vi "getWifiMode.vi"(8 "error":errorcluster, 11 "connection ID":refnum<k5>) -> (0 "error out":errorcluster, 2 "mode":i32, 3 "connection ID out":refnum<k5>)   [LabVIEW 2016, in "amc_api.lvlib"]
doc: "Gets the operation mode of the WiFi adapter."
uses:
  amc_api.lvlib
panel:
  out "jsonRespIn":string
  out "JSON-response":string="{\"jsonrpc\":\"2.0\",\"method\":\"\",\"params\":[5,1.245,true,\"name\"],\"id\":\"1\"}"
  out "JSON request":string
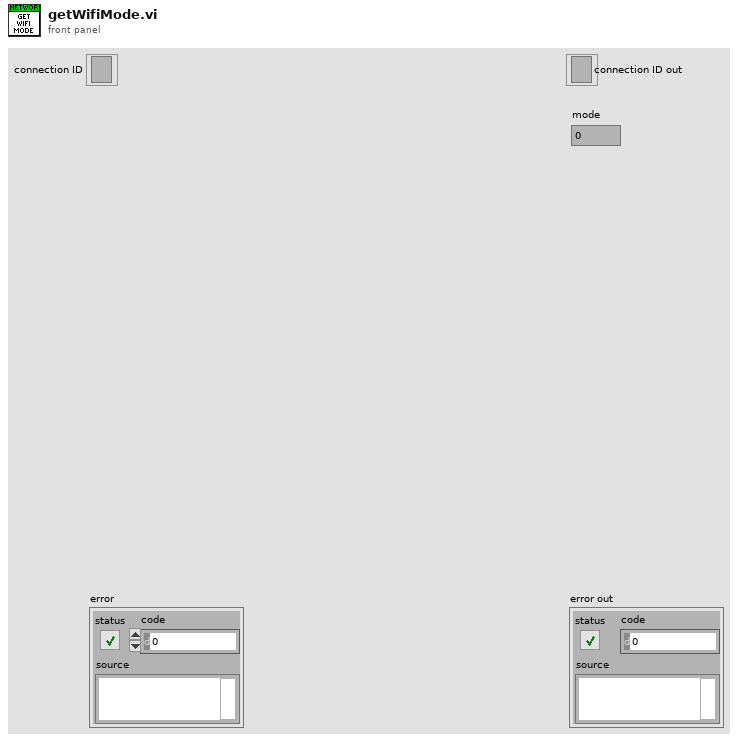
[diagram p1: front panel]
types:
  T1 = cluster{"jsonrpc":string, "method":string, "params":string[], "id":string, "api":i32, "pid":string}
  T2 = enum16{"Standard", "Buffered", "CRLF", "Immediate"}
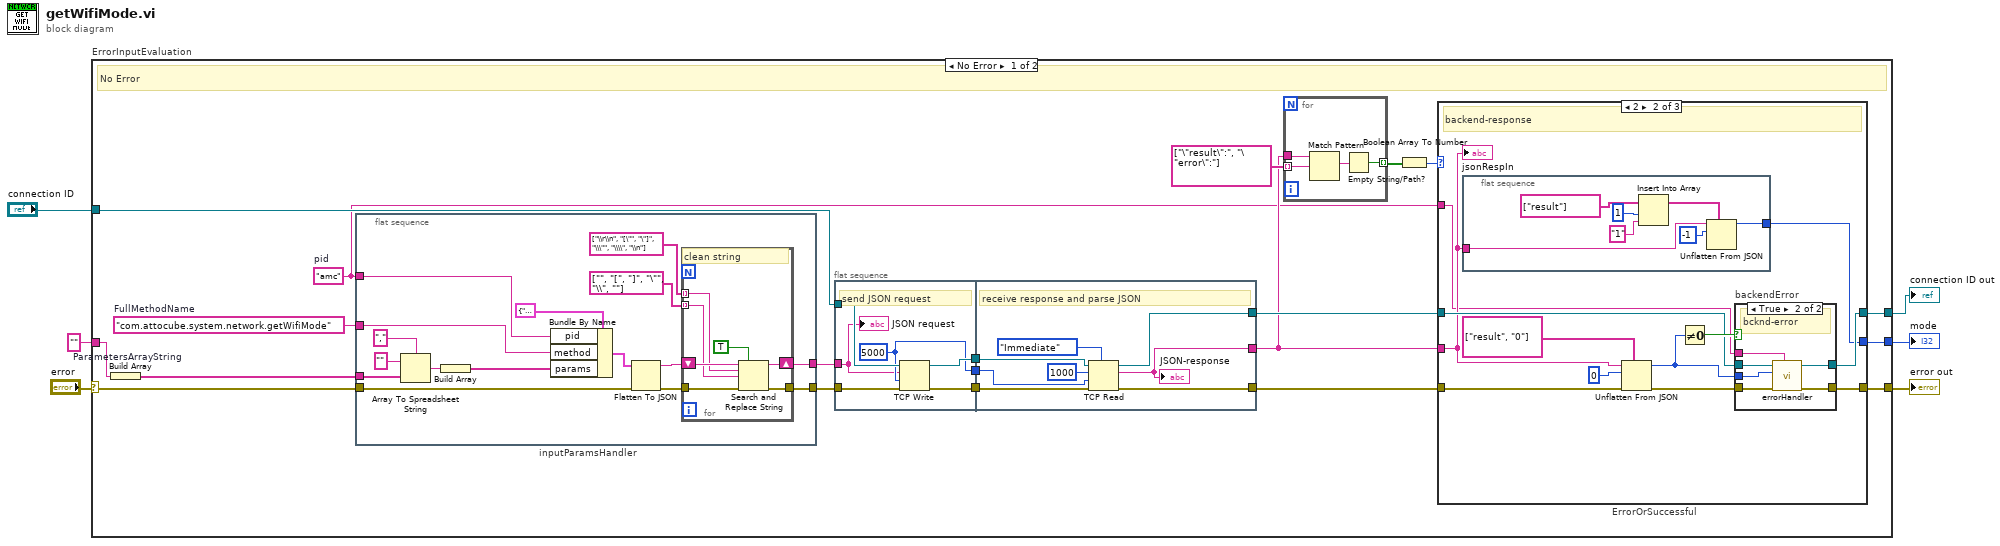
[diagram p0: block diagram]
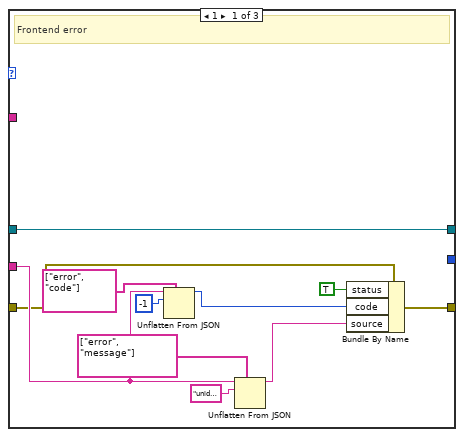
[diagram p2: hidden frame]
diagram:
  n1 = case "ErrorInputEvaluation" shown="No Error" "error" {
    selector: "error" -> [w13 w108]
    tunnel: "connection ID" -> [w23 w109]
    tunnel: [w15 w108] -> w5
    tunnel: [w16 w109] -> w4
    tunnel: "" -> [w8 _]
    tunnel: [w7 _] -> w1
    frame No Error {
      w9 = "amc"  # pid
      w14 = "com.attocube.system.network.getWifiMode"  # FullMethodName
      # "No Error"
      n2 = Build Array "ParametersArrayString"(w8) -> (w12:string[])
      n3 = flat-sequence "inputParamsHandler" {
        tunnel: [w32] -> w11
        tunnel: w12 -> [w38]
        tunnel: w13 -> [w37]
        tunnel: [w34] -> w10
        tunnel: w14 -> [w28]
        tunnel: w9 -> [w27]
        frame #0 {
          n4 = Array To Spreadsheet String(delimiter (Tab)=",", array=w38, 3:"" ("format string")) -> (spreadsheet string=w40:string)
          n5 = Build Array "Build Array"(w40) -> (w29:string[])
          n6 = Bundle By Name(cluster=T1 {"jsonrpc"="2.0", "method"="com.attocube.amc.res.setRESReadOutFreq", "params"=[], "id"="1", "api"=2, "pid"=""}, "pid"=w27, "method"=w28, "params"=w29) -> (w39:T1)
          n7 = Flatten To JSON(anything=w39, error in (no error)=w37) -> (JSON string=w33:string, 11:w35:errorcluster)  [unwired: 1 in]
          n8 = for {
            tunnel: string[] ["\\r\\n", "[\"", "\"]", "\\\"", "\\\\", "\\n"] ("search string") -> [w46] mode=indexing
            tunnel: string[] ["", "[", "]", "\"", "\\", ""] ("replace string (\"\")") -> [w45] mode=indexing
            shift-right: [w48] -> w32
            shift-left: w33 -> [w47]
            tunnel: w35 -> [w44]
            tunnel: [w43] -> w34
            # "clean string"
            n9 = Search and Replace String(replace all?=TRUE ("replace all? (F)"), input string=w47, search string=w46, replace string=w45, error in=w44) -> (result string=w48:string, error out=w43:errorcluster)  [unwired: 3 in, 2 out]
          }
        }
      }
      n10 = flat-sequence {
        tunnel: w23 -> [w99]
        tunnel: [w97] -> w26
        tunnel: [w98] -> w25
        tunnel: w10 -> [w94]
        tunnel: [w96] -> w24
        tunnel: w11 -> [w95]
        tunnel: [w103] -> w19
        tunnel: w26 -> [w105]
        tunnel: w25 -> [w104]
        tunnel: [w101] -> w18
        tunnel: w24 -> [w102]
        tunnel: [w100] -> w17
        frame #0 {
          w96 = 5000 ("timeout ms (25000)")
          # "send JSON request"
          n11 = TCP Write(connection ID=w99, data in=w95, error in (no error)=w94, 9:w96) -> (connection ID out=w97:refnum<k5>, error out=w98:errorcluster)  [unwired: 1 out]
          "JSON request" <- w95
        }
        frame #1 {
          # "receive response and parse JSON"
          n12 = TCP Read(connection ID=w105, bytes to read=1000, error in (no error)=w104, 7:T2."Immediate" ("mode (standard)"), 9:w102) -> (connection ID out=w103:refnum<k5>, data out=w100:string, error out=w101:errorcluster)
          "JSON-response" <- w100
        }
      }
      n13 = for {
        tunnel: string[] ["\"result\":", "\"error\":"] ("path") -> [w52] mode=indexing
        tunnel: [w50] -> w21 mode=indexing
        tunnel: w17 -> [w53]
        n14 = Match Pattern(string=w53, regular expression=w52) -> (match substring=w51:string)  [unwired: 1 in, 3 out]
        n15 = Empty String/Path?(string/path=w51) -> (empty?=w50:bool)
      }
      n16 = Boolean Array To Number(Boolean array=w21) -> (number=w20:u32)
      n17 = case "ErrorOrSuccessful" shown="2" w20 {
        tunnel: w17 -> [w56 w67 _]
        tunnel: w19 -> [w54 w70 w93]
        tunnel: [w54 w69 w93] -> w16
        tunnel: [w57 w68 w92] -> w15
        tunnel: w18 -> [w55 w71 w92]
        tunnel: w9 -> [_ w66 _]
        tunnel: [_ w65 _] -> w7
        frame 1 {
          # "Frontend error"
          n18 = Unflatten From JSON(path=string[] ["error", "code"], JSON string=w56, type and defaults=-1) -> (value=w63:i32)  [unwired: 4 in, 1 out]
          n19 = Unflatten From JSON(path=string[] ["error", "message"], JSON string=w56, type and defaults="unidentified error") -> (value=w64:string)  [unwired: 4 in, 1 out]
          n20 = Bundle By Name(cluster=w55, "status"=TRUE, "code"=w63, "source"=w64) -> (w57:errorcluster)
        }
        frame 2 {
          # "backend-response"
          n21 = flat-sequence "out_integer" {
            tunnel: w67 -> [w79]
            tunnel: [w77] -> w65
            frame #0 {
              n22 = Insert Into Array(array=string[] ["result"] ("path"), index=1, new element="1" ("idx")) -> (w81:string[])
              n23 = Unflatten From JSON(path=w81, JSON string=w79, type and defaults=-1 ("index")) -> (value=w77:i32)  [unwired: 4 in, 1 out]
            }
          }
          n24 = Unflatten From JSON(path=string[] ["result", "0"], JSON string=w67, type and defaults=0, error in (no error)=w71) -> (value=w76:i32, error out=w74:errorcluster)  [unwired: 3 in]
          n25 = Not Equal To 0?(x=w76) -> (x != 0?=w75:bool)
          n26 = case "backendError" shown="True" w75 {
            tunnel: w76 -> [_ w91]
            tunnel: w74 -> [w85 w90]
            tunnel: [w84 w89] -> w69
            tunnel: [w85 w88] -> w68
            tunnel: w70 -> [w84 w87]
            tunnel: w66 -> [_ w86]
            frame False {
              # "successful"
            }
            frame True {
              # "bcknd-error"
              n27 = call "errorHandler.vi"("pid"=w86, "error in"=w90, "errNbr"=w91, "connection ID"=w87) -> ("error out 2"=w88:errorcluster, "connection ID out"=w89:refnum<k5>)  [unwired: 6 in]
            }
          }
          "jsonRespIn" <- w67
        }
        frame Default {
          # "NoResponse"
        }
      }
    }
    frame Error {
      # "Error"
    }
  }
  "error out" <- w5
  "connection ID out" <- w4
  "mode" <- w1
